vi "TcpCommunication.vi"(1 "Address":string="localhost", 2 "Port":u16=38300) -> ()   [LabVIEW 2013]
panel:
  in  "Delay":u32=350
  in  "Continue?":bool
  in  "Command":string="00"
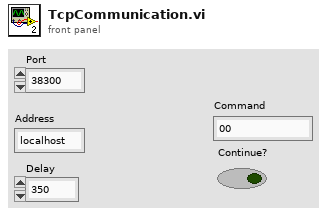
[diagram p1: front panel]
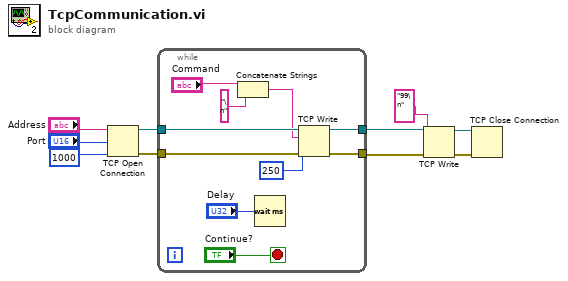
[diagram p0: block diagram]
diagram:
  n1 = TCP Open Connection(address="Address", remote port or service name="Port", timeout ms (60000)=1000) -> (connection ID=w6:refnum<k5>, error out=w7:errorcluster)  [unwired: 2 in]
  n2 = while {
    tunnel: w7 -> [w20]
    tunnel: w6 -> [w19]
    tunnel: [w17] -> w2
    tunnel: [w16] -> w1
    stop <- "Continue?" stop-if-true
    n3 = Concatenate Strings("Command", "\n" ("string")) -> (w12:string)
    n4 = Wait (ms)(milliseconds to wait="Delay") -> ()  [unwired: 1 out]
    n5 = TCP Write(connection ID=w19, data in=w12, error in (no error)=w20, 9:250 ("timeout ms (25000)")) -> (connection ID out=w17:refnum<k5>, error out=w16:errorcluster)  [unwired: 1 out]
  }
  n6 = TCP Write(connection ID=w2, data in="99\n", error in (no error)=w1) -> (connection ID out=w5:refnum<k5>, error out=w4:errorcluster)  [unwired: 1 in, 1 out]
  n7 = TCP Close Connection(connection ID=w5, error in (no error)=w4) -> ()  [unwired: 1 in, 2 out]
